vi "Generate_WayPoints_ConstantDistanceNOREVERSE_dualVcontrol.vi"(5 "Update Position Loop Wait Time (us)":u32=50000, 11 "Input Cluster":T2={"Scan Rate (um/s)"=15.0, "X Start"=15.0, "X End"=15.0, "Y Start"=15.0, "Y End"=15.0, " Z Start"=15.0, "Number of Lines"=15, "V"=15.0, "Z End"=15.0, "Approach Rate (um/s)"=15.0, "HoldTime / s"=15, "Scan V1"=15.0, "Retract V1"=15.0, "Approach V2"=15.0, "Scan V2"=15.0, "Retract V2"=15.0}) -> (0 "output cluster":T1)   [LabVIEW 2023]
uses:
  TypeDefs/WayPointCluster.ctl
  User_Vi/Settings.vi
panel:
  out "X Current":dbl
  in  "WayPointCluster":T1
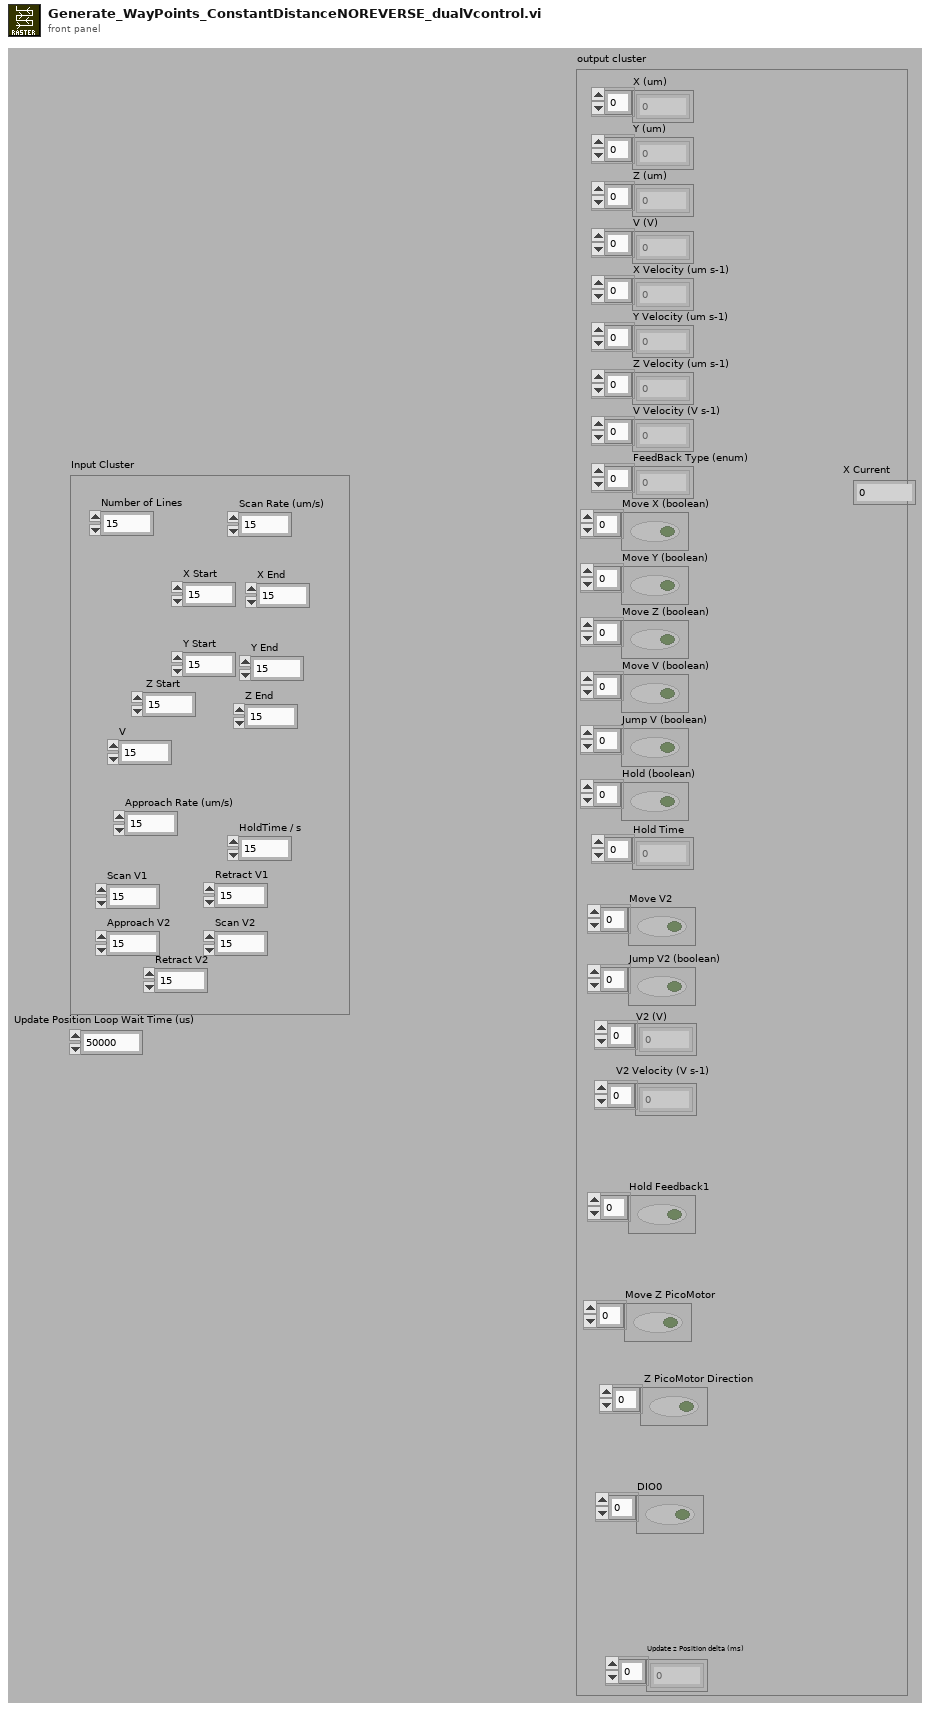
[diagram p1: front panel]
types:
  T1 = typedef "WayPointCluster.ctl" = cluster{"X (um)":dbl[], "Y (um)":dbl[], "Z (um)":dbl[], "V (V)":dbl[], "X Velocity (um s-1)":dbl[], "Y Velocity (um s-1)":dbl[], "Z Velocity (um s-1)":dbl[], "V Velocity (V s-1)":dbl[], "FeedBack Type (enum)":u16[], "Move X (boolean)":bool[], "Move Y (boolean)":bool[], "Move Z (boolean)":bool[], "Move V (boolean)":bool[], "Jump V (boolean)":bool[], "Hold (boolean)":bool[], "Hold Time":u32[], "V2 (V)":dbl[], "Move V2":bool[], "V2 Velocity (V s-1)":dbl[], "Jump V2 (boolean)":bool[], "Update z Position delta (ms)":i16[], "Hold Feedback1":bool[], "Move Z PicoMotor":bool[], " Z PicoMotor Direction":bool[], "DIO0":bool[]}
  T2 = cluster{"Scan Rate (um/s)":dbl, "X Start":dbl, "X End":dbl, "Y Start":dbl, "Y End":dbl, " Z Start":dbl, "Number of Lines":u32, "V":dbl, "Z End":dbl, "Approach Rate (um/s)":dbl, "HoldTime / s":u32, "Scan V1":dbl, "Retract V1":dbl, "Approach V2":dbl, "Scan V2":dbl, "Retract V2":dbl}
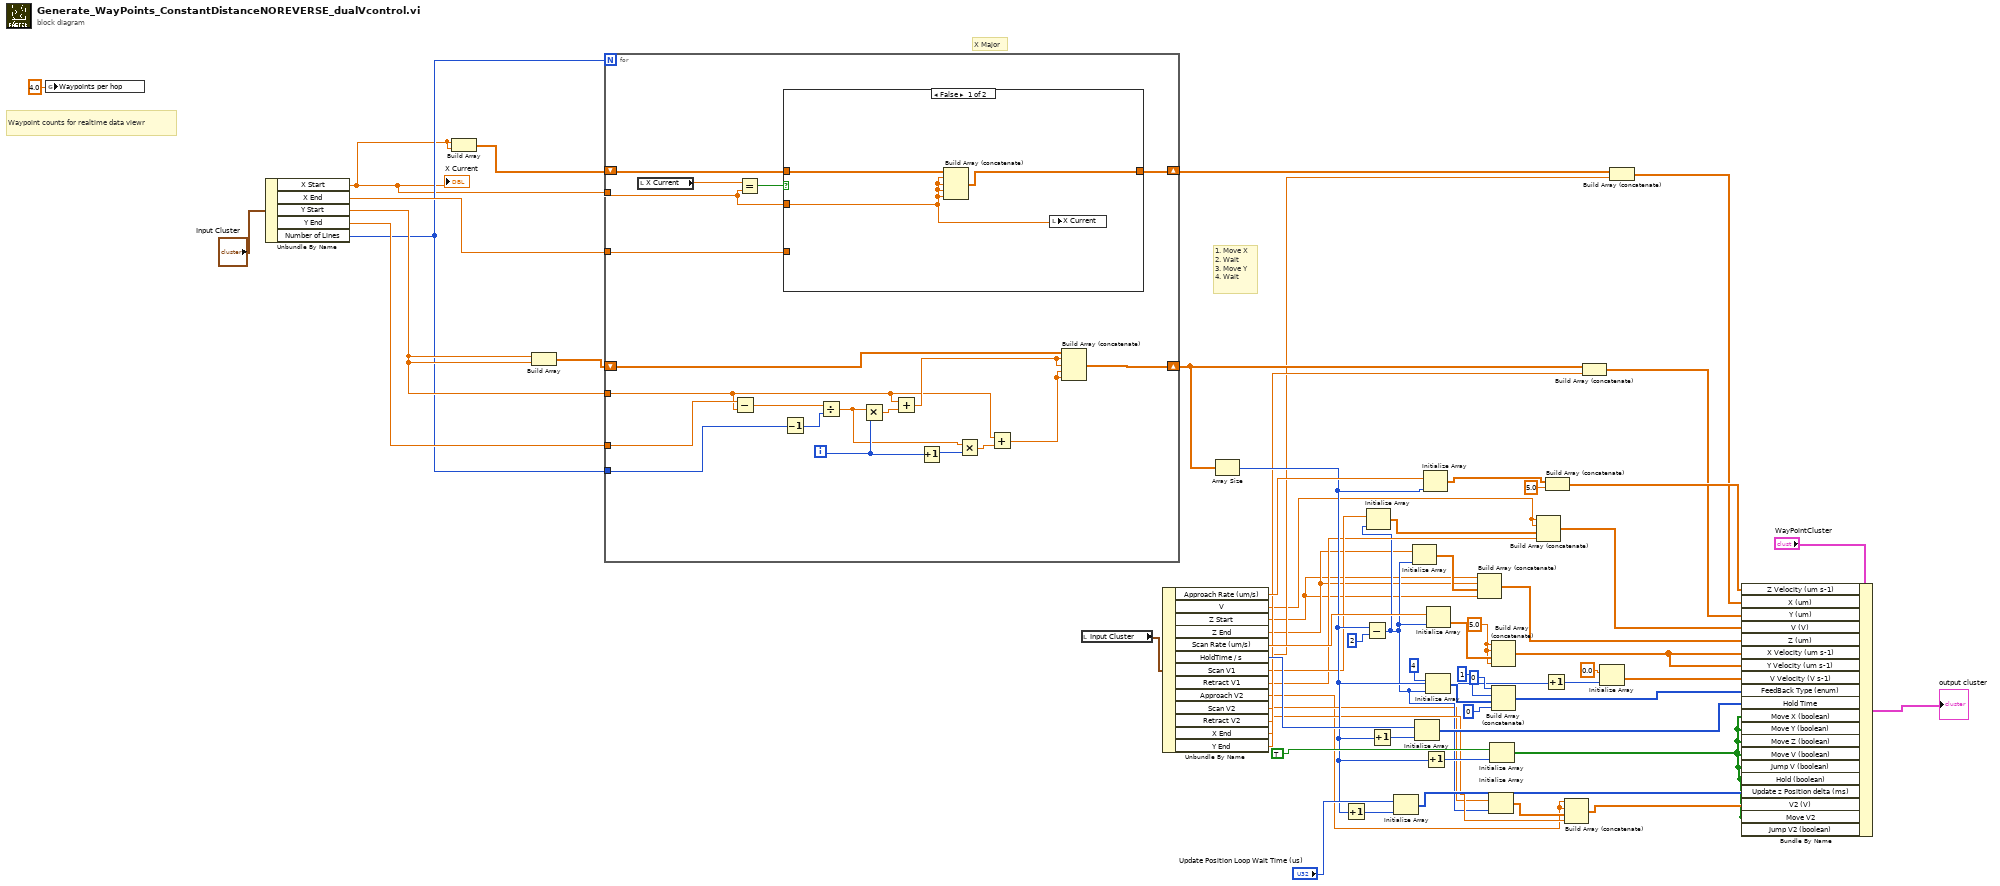
[diagram p0: block diagram]
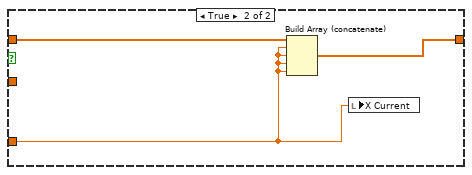
[diagram p2: hidden frame]
diagram:
  w15 = 5.0 ("element")
  # "Waypoint counts for realtime data viewr"
  # "1. Move X\n2. Wait\n3. Move Y\n4. Wait"
  # "X Major"
  n1 = global write "Settings.vi" "Waypoints per hop"(4.0 ("Waypoints per hop")) -> ()
  n2 = Unbundle By Name("Input Cluster") -> ("X Start"=w33:dbl, "X End"=w36:dbl, "Y Start"=w35:dbl, "Y End"=w60:dbl, "Number of Lines"=w34:u32)
  "X Current" <- w33
  n3 = Build Array(w33, w33) -> (w37:dbl[])
  n4 = Build Array(w35, w35) -> (w38:dbl[])
  n5 = for {
    N: w34 -> [_]
    tunnel: w60 -> [w81]
    tunnel: w34 -> [w78]
    shift-right: [w73] -> w24
    shift-left: w38 -> [w77]
    shift-right: [w74] -> w21
    shift-left: w37 -> [w76]
    tunnel: w36 -> [w72]
    tunnel: w35 -> [w64]
    tunnel: w33 -> [w62]
    i -> [w68]
    n6 = local read "X Current"() -> (w69:dbl)
    n7 = Subtract(x=w81, y=w64) -> (x-y=w80:dbl)
    n8 = Equal?(x=w69, y=w62) -> (x = y?=w70:bool)
    n9 = case shown="False" w70 {
      tunnel: w76 -> [w83 w87]
      tunnel: [w84 w86] -> w74
      tunnel: w72 -> [_ w85]
      tunnel: w62 -> [w82 _]
      frame False {
        n10 = Build Array (concatenate)(w83, w82, w82, w82, w82) -> (w84:dbl[])
        n11 = local write "X Current"(w82) -> ()
      }
      frame True {
        n12 = Build Array (concatenate)(w87, w85, w85, w85, w85) -> (w86:dbl[])
        n13 = local write "X Current"(w85) -> ()
      }
    }
    n14 = Decrement(x=w78) -> (x-1=w75:u32)
    n15 = Divide(x=w80, y=w75) -> (x/y=w65:dbl)
    n16 = Multiply(x=w65, y=w68) -> (x*y=w79:dbl)
    n17 = Add(x=w64, y=w79) -> (x+y=w71:dbl)
    n18 = Increment(x=w68) -> (x+1=w66:i32)
    n19 = Multiply(x=w65, y=w66) -> (x*y=w67:dbl)
    n20 = Add(x=w64, y=w67) -> (x+y=w63:dbl)
    n21 = Build Array (concatenate)(w77, w71, w71, w63, w63) -> (w73:dbl[])
  }
  n22 = local read "Input Cluster"() -> (w58:T2)
  n23 = Unbundle By Name(w58) -> ("Approach Rate (um/s)"=w32:dbl, "V"=w18:dbl, "Z Start"=w1:dbl, "Z End"=w2:dbl, "Scan Rate (um/s)"=w51:dbl, "HoldTime / s"=w57:u32, "Scan V1"=w17:dbl, "Retract V1"=w16:dbl, "Approach V2"=w5:dbl, "Scan V2"=w7:dbl, "Retract V2"=w9:dbl, "X End"=w22:dbl, "Y End"=w25:dbl)
  n24 = Array Size(array=w24) -> (size(s)=w31:i32)
  n25 = Increment(x=w31) -> (x+1=w10:i32)
  n26 = Subtract(x=w31, y=2) -> (x-y=w8:i32)
  n27 = Initialize Array(w17, w8) -> (w19:dbl[])
  n28 = Increment(x=w31) -> (x+1=w12:i32)
  n29 = Initialize Array("Update Position Loop Wait Time (us)", w10) -> (w39:u32[])
  n30 = Initialize Array(w2, w8) -> (w42:dbl[])
  n31 = Initialize Array(w57, w12) -> (w52:u32[])
  n32 = Initialize Array(w32, w31) -> (w27:dbl[])
  n33 = Increment(x=w31) -> (x+1=w11:i32)
  n34 = Initialize Array(u32 4 ("element"), w8) -> (w44:u32[])
  n35 = Initialize Array(w51, w8) -> (w48:dbl[])
  n36 = Build Array (concatenate)(w1, w2, w42, w1) -> (w41:dbl[])
  n37 = Initialize Array(w7, w8) -> (w6:dbl[])
  n38 = Initialize Array(TRUE, w11) -> (w3:bool[])
  n39 = Build Array (concatenate)(w15, w15, w48, w15) -> (w49:dbl[])
  n40 = Build Array (concatenate)(u32 0 ("element"), u32 1 ("element"), w44, u32 0 ("element")) -> (w43:u32[])
  n41 = Build Array (concatenate)(w18, w18, w19, w16) -> (w20:dbl[])
  n42 = Increment(x=w31) -> (x+1=w14:i32)
  n43 = Build Array (concatenate)(w27, 5.0 ("element")) -> (w29:dbl[])
  n44 = Build Array (concatenate)(w5, w5, w6, w9) -> (w4:dbl[])
  n45 = Build Array (concatenate)(w24, w25) -> (w26:dbl[])
  n46 = Initialize Array(0.0 ("element"), w14) -> (w53:dbl[])
  n47 = Build Array (concatenate)(w21, w22) -> (w23:dbl[])
  n48 = Bundle By Name(cluster="WayPointCluster", "Z Velocity (um s-1)"=w29, "X (um)"=w23, "Y (um)"=w26, "V (V)"=w20, "Z (um)"=w41, "X Velocity (um s-1)"=w49, "Y Velocity (um s-1)"=w49, "V Velocity (V s-1)"=w53, "FeedBack Type (enum)"=w43, "Hold Time"=w52, "Move X (boolean)"=w3, "Move Y (boolean)"=w3, "Move Z (boolean)"=w3, "Move V (boolean)"=w3, "Jump V (boolean)"=w3, "Hold (boolean)"=w3, "Update z Position delta (ms)"=w39, "V2 (V)"=w4, "Move V2"=w3, "Jump V2 (boolean)"=w3) -> (→"output cluster":T1)
